vi "GetSpeed1.vi"() -> (3 "Characters Read 3":string)   [LabVIEW 2015]
uses:
  <vilib>/myRIO/Instrument Drivers/Onboard IO/UART/typedef/VISA Configuration.ctl
  <vilib>/Instr/_visa.llb/VISA Configure Serial Port (Instr).vi
  <vilib>/myRIO/Express VI/Onboard IO/UART/UART Express VI.xnode
  <vilib>/myRIO/Instrument Drivers/Onboard IO/UART/UART.lvlib
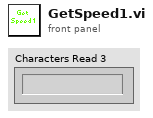
[diagram p1: front panel]
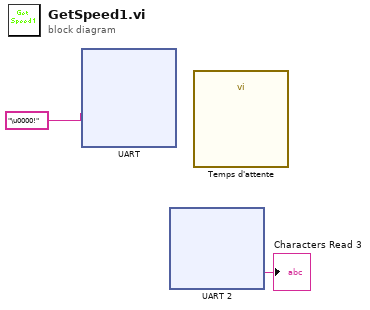
[diagram p0: block diagram]
diagram:
  n1 = xnode "UART"("Characters to Write"="\u0000!") -> ()  [unwired: 1 in, 2 out]
  n2 = xnode "UART 2"() -> ("Characters Read"=→"Characters Read 3":string)  [unwired: 1 in, 1 out]
  n3 = call "Temps d'attente"() -> ()  [unwired: 11 in, 1 out]
